vi "GD and kalibration Infos.vi"(11 "Sprachliste":string[][](array[string])) -> (0 "Error occured":bool, 2 "ErrorMessage PDF":string, 3 "ErrorMessages LogFile":string, 4 "ErrorMessage Kalibrieren PDF":string, 6 "ErrorMessage GD PDF":string)   [LabVIEW 2020, in "Linearisierung v2.lvlib" / "Protokoll.lvlib"]
uses:
  Protokoll.lvlib
  SpanEinstellungen/SpanEinstellungen.lvlib
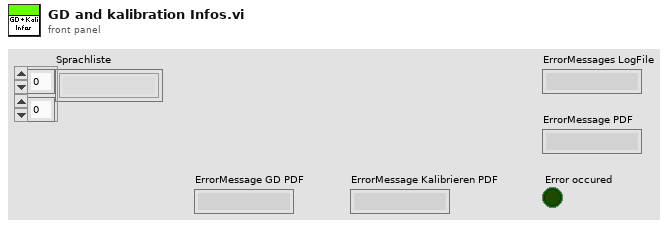
[diagram p1: front panel]
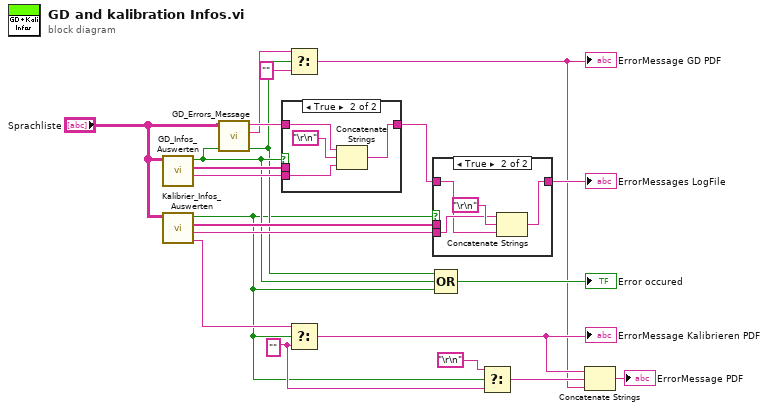
[diagram p0: block diagram]
diagram:
  w8 = "" ("f")
  n1 = call "GD_Infos_Auswerten.vi"("Sprachliste"="Sprachliste") -> ("GD Info Text"=w18:string, "GD Infos Array"=w20:string[], "GD Error occured"=w13:bool)  [unwired: 8 in]
  n2 = call "Kalibrier_Infos_Auswerten.vi"("Sprachliste"="Sprachliste") -> ("ErrorMessage PDF"=w10:string, "Kalibrier Info Text"=w17:string, "Kalibrier Infos Array"=w19:string[], "Kalibrier Error occured"=w2:bool)  [unwired: 7 in]
  n3 = call "GD_Errors_Message.vi"("Errors woanders in"=w13, "Sprachliste"="Sprachliste") -> ("Errors"=w7:bool, "ErrorMessage PDF"=w12:string, "ErrorMessages LogFile"=w21:string)  [unwired: 7 in]
  n4 = case shown="True" w13 {
    tunnel: w21 -> [w22 w26]
    tunnel: [w22 w23] -> w3
    tunnel: w20 -> [_ _]
    tunnel: w18 -> [_ w24]
    frame False {
    }
    frame True {
      n5 = Concatenate Strings(w26, "\r\n", w24) -> (w23:string)
    }
  }
  n6 = Select(t=w12, s=w7, f="") -> (s? t:f=w1:string)
  "ErrorMessage GD PDF" <- w1
  n7 = Select(t=w10, s=w2, f=w8) -> (s? t:f=w5:string)
  "ErrorMessage Kalibrieren PDF" <- w5
  n8 = case shown="True" w2 {
    tunnel: w3 -> [w27 w28]
    tunnel: [w27 w30] -> w15
    tunnel: w19 -> [_ _]
    tunnel: w17 -> [_ w29]
    frame False {
    }
    frame True {
      n9 = Concatenate Strings(w29, "\r\n", w28) -> (w30:string)
    }
  }
  "ErrorMessages LogFile" <- w15
  n10 = Compound Arithmetic op=OR ("Mehrfacharithmetik")(w7, w13, w2) -> (→"Error occured":bool)
  n11 = Select(t="\r\n", s=w2, f=w8) -> (s? t:f=w4:string)
  n12 = Concatenate Strings(w5, w4, w1) -> (→"ErrorMessage PDF":string)
